vi "NDAP_ver6-16_zZQuickFix.vi"() -> ()   [LabVIEW 2013]
panel:
  out "file path":path
  out "Is recording data":bool
  in  "stop (F)":bool
  in  "Intercepts":dbl[](array[numeric])
  in  "Slopes":dbl[](array[numeric])
  in  "Tab Control":T1(tab)
  out "PT 1":dbl[](graph)
  out "PT 2":dbl[](graph)
  out "PT 4":dbl[](graph)
  out "PT 3":dbl[](graph)
  out "PT 5":dbl[](graph)
  out "PT 6":dbl[](graph)
  out "PT 7":dbl[](graph)
  out "PT 8":dbl[](graph)
  out "LC 2-1":dbl[](graph)
  out "LC 1":dbl[](graph)
  out "LC 2":dbl[](graph)
  out "FM":dbl[](graph)
  out "TC 1":dbl[](graph)
  out "TC 2":dbl[](graph)
  out "TC 3":dbl[](graph)
  out "TC 4":dbl[](graph)
  # "Slope must be 1 and Intercepts\nmust be 0 (not greyed out)\nfor this to work"
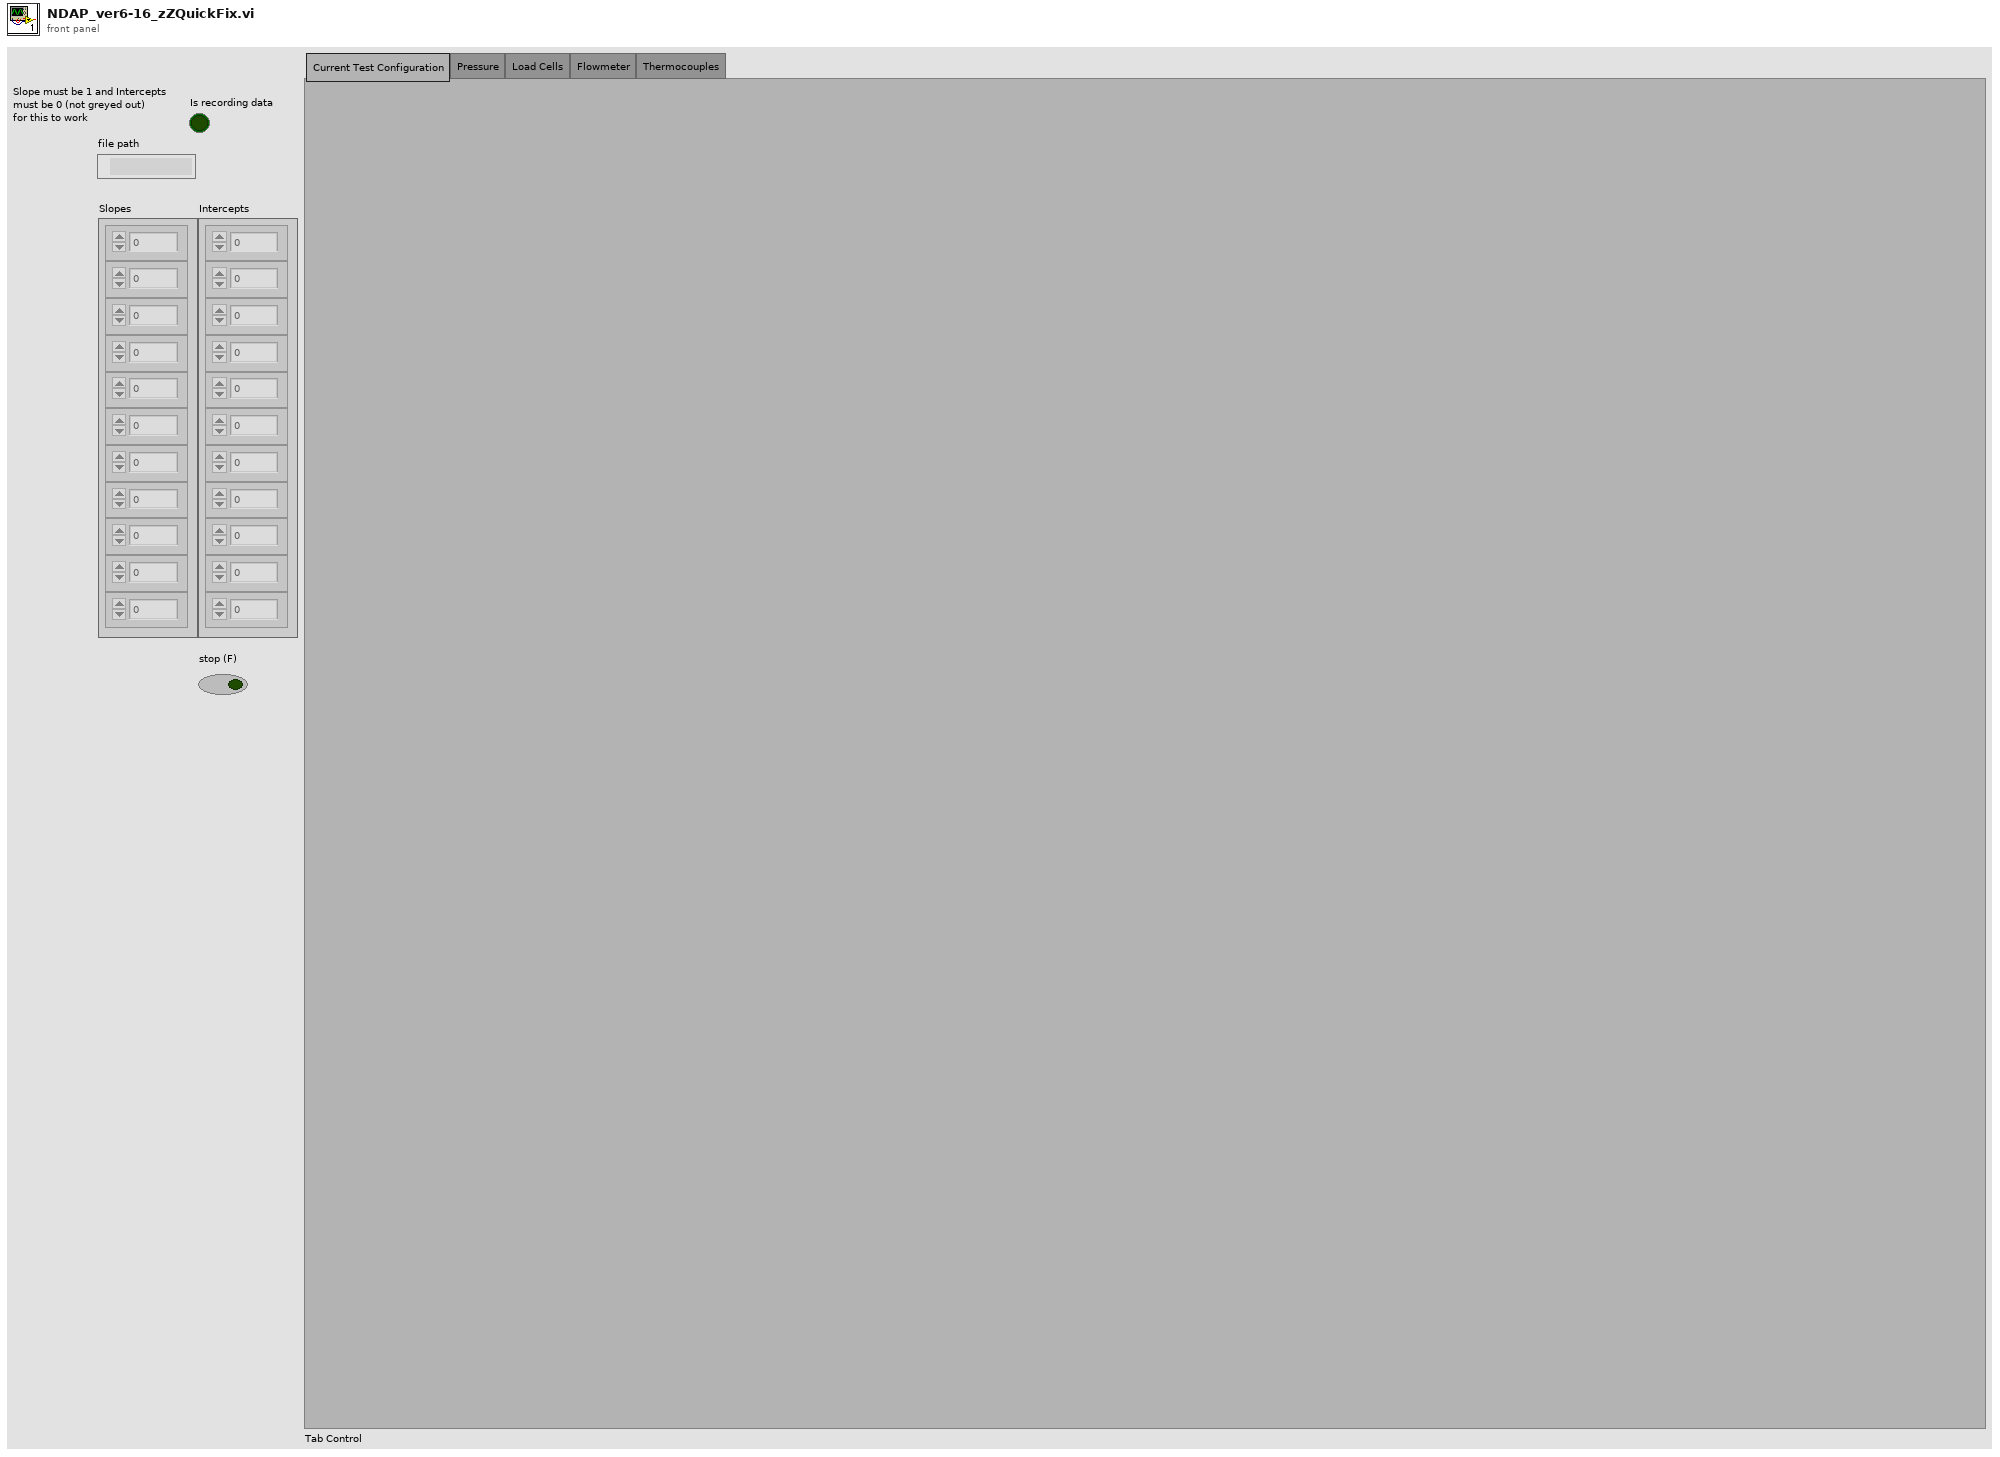
[diagram p1: front panel]
types:
  T1 = enum32{"Current Test Configuration", "Pressure", "Load Cells", "Flowmeter", "Thermocouples"}
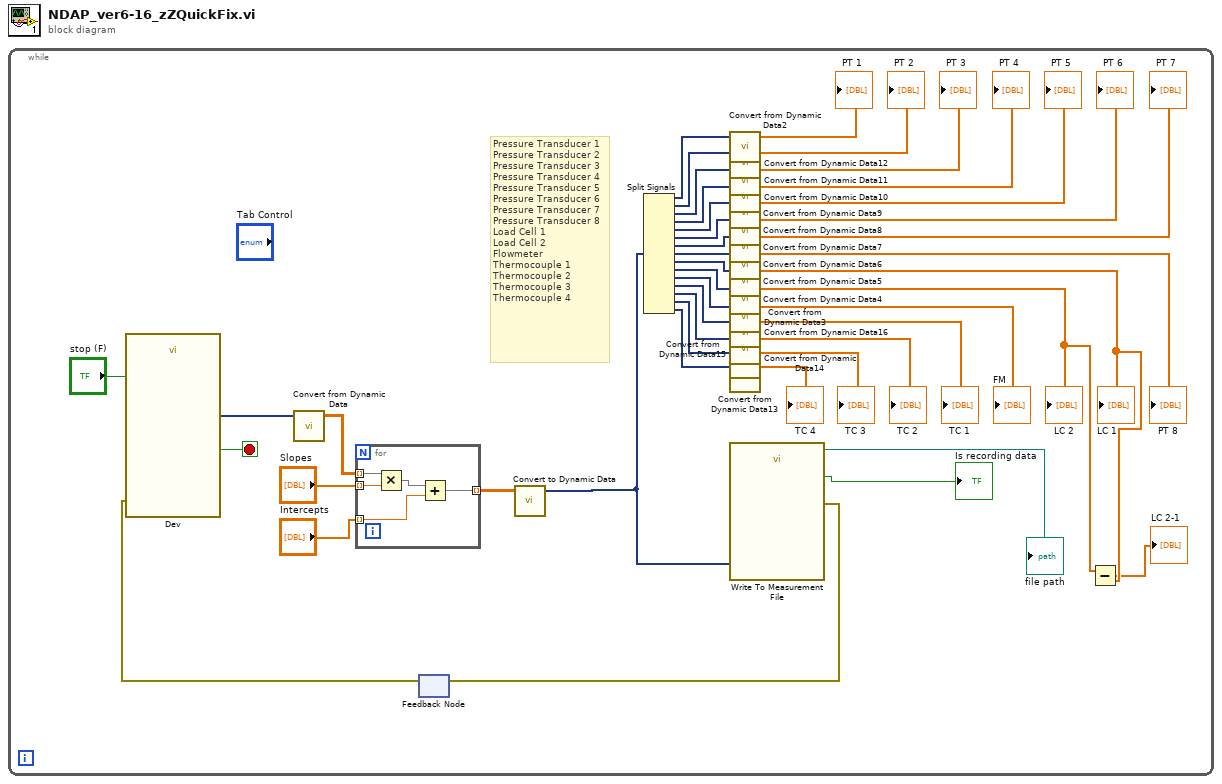
[diagram p0: block diagram]
diagram:
  n1 = while {
    stop <- w42 stop-if-true
    # "Pressure Transducer 1\nPressure Transducer 2\nPressure Transducer 3\nPressure Transducer 4\nPressure Transducer 5\nPressure Transducer 6\nPressure Transducer 7\nPressure Transducer 8\nLoad Cell 1\nLoad Cell 2\nFlowmeter\nThermocouple 1\nThermocouple 2\nThermocouple 3\nThermocouple 4"
    n2 = feedback #1() -> (w35:errorcluster)  [unwired: 1 in]
    n3 = call "Dev"("error in"=w35, "stop (F)"="stop (F)") -> ("data"=w41:dynamicdata, "stopped"=w42:bool)  [unwired: 14 in, 2 out]
    n4 = call "Convert from Dynamic Data"("Dynamic Data Type"=w41) -> ("Array"=w38:dbl[][])  [unwired: 3 in]
    n5 = for {
      tunnel: w38 -> [w48] mode=indexing
      tunnel: "Slopes" -> [w47] mode=indexing
      tunnel: "Intercepts" -> [w45] mode=indexing
      tunnel: [w44] -> w37 mode=indexing
      n6 = Multiply(x=w48, y=w47) -> (x*y=w46:dbl[])
      n7 = Add(x=w46, y=w45) -> (x+y=w44:dbl[])
    }
    n8 = call "Convert to Dynamic Data"("2D Array"=w37) -> ("Dynamic Data Type"=w6:dynamicdata)  [unwired: 3 in]
    n9 = Split Signals(w6) -> (w34:dynamicdata, w32:dynamicdata, w30:dynamicdata, w28:dynamicdata, w26:dynamicdata, w24:dynamicdata, w22:dynamicdata, w20:dynamicdata, w18:dynamicdata, w17:dynamicdata, w16:dynamicdata, w14:dynamicdata, w12:dynamicdata, w10:dynamicdata, w8:dynamicdata)  [unwired: 15 in]
    n10 = call "Convert from Dynamic Data2"("Dynamic Data Type"=w34) -> ("Array"=→"PT 1":dbl[])  [unwired: 3 in]
    n11 = call "Convert from Dynamic Data12"("Dynamic Data Type"=w32) -> ("Array"=→"PT 2":dbl[])  [unwired: 3 in]
    n12 = call "Convert from Dynamic Data11"("Dynamic Data Type"=w30) -> ("Array"=→"PT 3":dbl[])  [unwired: 3 in]
    n13 = call "Convert from Dynamic Data10"("Dynamic Data Type"=w28) -> ("Array"=→"PT 4":dbl[])  [unwired: 3 in]
    n14 = call "Convert from Dynamic Data9"("Dynamic Data Type"=w26) -> ("Array"=→"PT 5":dbl[])  [unwired: 3 in]
    n15 = call "Convert from Dynamic Data8"("Dynamic Data Type"=w24) -> ("Array"=→"PT 6":dbl[])  [unwired: 3 in]
    n16 = call "Convert from Dynamic Data7"("Dynamic Data Type"=w22) -> ("Array"=→"PT 7":dbl[])  [unwired: 3 in]
    n17 = call "Convert from Dynamic Data6"("Dynamic Data Type"=w20) -> ("Array"=→"PT 8":dbl[])  [unwired: 3 in]
    n18 = call "Convert from Dynamic Data5"("Dynamic Data Type"=w18) -> ("Array"=w3:dbl[])  [unwired: 3 in]
    "LC 1" <- w3
    n19 = call "Convert from Dynamic Data4"("Dynamic Data Type"=w17) -> ("Array"=w2:dbl[])  [unwired: 3 in]
    "LC 2" <- w2
    n20 = call "Convert from Dynamic Data3"("Dynamic Data Type"=w16) -> ("Array"=→"FM":dbl[])  [unwired: 3 in]
    n21 = call "Convert from Dynamic Data16"("Dynamic Data Type"=w14) -> ("Array"=→"TC 1":dbl[])  [unwired: 3 in]
    n22 = call "Convert from Dynamic Data15"("Dynamic Data Type"=w12) -> ("Array"=→"TC 2":dbl[])  [unwired: 3 in]
    n23 = call "Convert from Dynamic Data14"("Dynamic Data Type"=w10) -> ("Array"=→"TC 3":dbl[])  [unwired: 3 in]
    n24 = call "Convert from Dynamic Data13"("Dynamic Data Type"=w8) -> ("Array"=→"TC 4":dbl[])  [unwired: 3 in]
    n25 = call "Write To Measurement File"("Signals"=w6) -> ("Filename Out"=→"file path":path, "Saving Data"=→"Is recording data":bool, "error out"=w36:errorcluster)  [unwired: 16 in]
    n26 = feedback-in #1(w36) -> ()
    n27 = Subtract(x=w2, y=w3) -> (x-y=→"LC 2-1":dbl[])
  }
